vi "destroy.vi"(8 "error in (no error)":errorcluster, 11 "simple_html_chat_ui in":refnum<class "simple_html_chat_ui.lvclass">) -> (0 "error out":errorcluster, 3 "simple_html_chat_ui out":refnum<class "simple_html_chat_ui.lvclass">)   [LabVIEW 2020, in "simple_html_chat_ui.lvclass"]
uses:
  simple_html_chat_ui.lvclass
  typedefs/ui_user_event.ctl
  simple_html_chat_ui.lvclass/simple_html_chat_ui.ctl
  WebSockets-API/Source/WebSockets/WebSocket Server/WebSocket Server.lvclass
  <vilib>/httpClient/LabVIEWHTTPClient.lvlib
  <vilib>/httpClient/POSTBuffer.vi
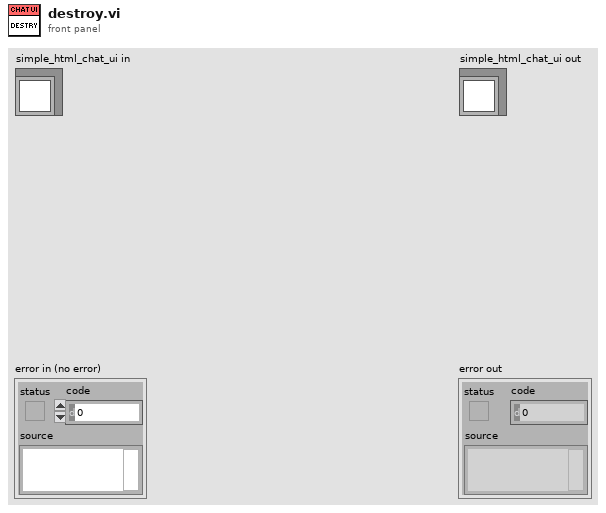
[diagram p1: front panel]
types:
  T1 = typedef "simple_html_chat_ui.lvclass/ui_user_event.ctl" = enum16{"Initialize", "Generate", "Get Reference", "Destroy"}
  T2 = typedef "LabVIEWHTTPClient.lvlib/ClientHandle.ctl" = refnum<k1>
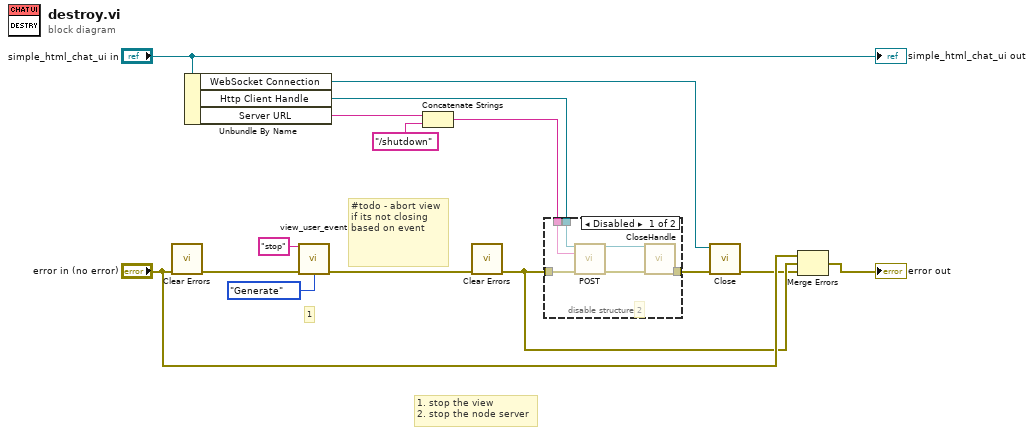
[diagram p0: block diagram]
diagram:
  # "#todo - abort view if its not closing based on event"
  # "1"
  # "1. stop the view\n2. stop the node server"
  n1 = call <vilib>:"Clear Errors.vi"("error in (no error)"="error in (no error)") -> ("error out"=w6:errorcluster)  [unwired: 5 in, 1 out]
  n2 = Unbundle By Name("simple_html_chat_ui in") -> ("WebSocket Connection"=w1:refnum<class "WebSocket Server.lvclass">, "Http Client Handle"=w13:T2, "Server URL"=w12:string)
  n3 = call "view_user_event.vi"("State"="stop", "error in (no error)"=w6, "Operation"=ui_user_event."Generate") -> ("error out"=w9:errorcluster)  [unwired: 11 in, 1 out]
  n4 = Concatenate Strings(w12, "/shutdown" ("string")) -> (w10:string)
  n5 = call <vilib>:"Clear Errors.vi"("error in (no error)"=w9) -> ("error out"=w3:errorcluster)  [unwired: 5 in, 1 out]
  n6 = disable-structure shown="Disabled" {
    disable-tunnel: [w21 w22] -> w15
    disable-tunnel: w13 -> [w18 _]
    disable-tunnel: w10 -> [w17 _]
    disable-tunnel: w3 -> [w16 w22]
    frame Disabled {
      # "2"
      n7 = call-poly <vilib>:"POST.vi"("client handle"=w18, "url"=w17, "error in (no error)"=w16) -> ("client handle out"=w19:T2, "error out"=w20:errorcluster)  [unwired: 9 in, 2 out]
      n8 = call <vilib>:"CloseHandle.vi"("client handle"=w19, "error in (no error)"=w20) -> ("error out"=w21:errorcluster)  [unwired: 13 in]
    }
    frame Enabled {
    }
  }
  n9 = call-dynamic "Close.vi"("error in (no error)"=w15, "WebSocket in"=w1) -> ("error out"=w2:errorcluster)  [unwired: 9 in]
  n10 = Merge Errors("error in (no error)", w3, w2) -> (→"error out":errorcluster)
  "simple_html_chat_ui out" <- "simple_html_chat_ui in"
